vi "ArrayInRunTIme.vi"() -> ()   [LabVIEW 2019]
panel:
  in  "Array 2":dbl[](array[numeric])
  out "appended array":dbl[](array[numeric])
  in  "c":dbl
  in  "b":dbl
  in  "a":dbl
  out "initialized array":dbl[](array[numeric])
  in  "Array":dbl[](array[numeric])
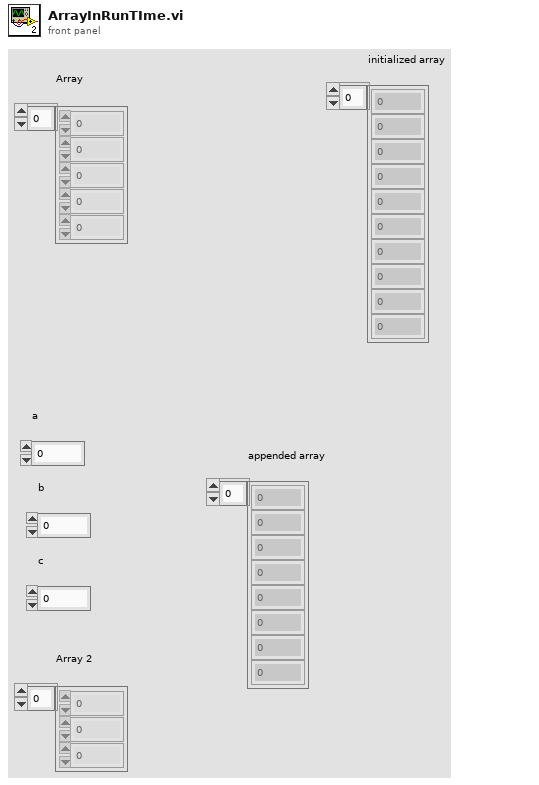
[diagram p1: front panel]
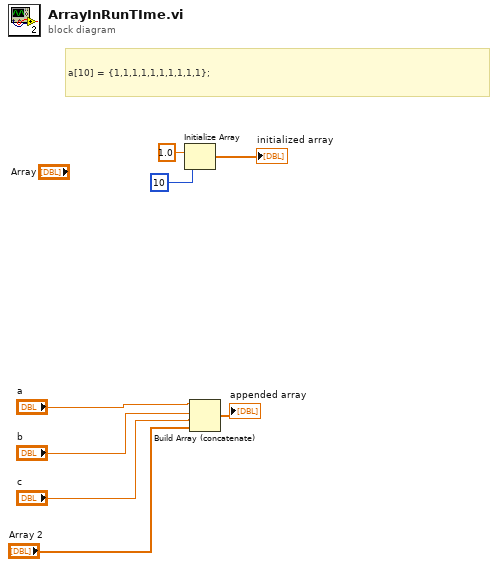
[diagram p0: block diagram]
diagram:
  # "a[10] = {1,1,1,1,1,1,1,1,1,1};"
  n1 = Initialize Array(1.0 ("element"), 10 ("dimension size")) -> (→"initialized array":dbl[])
  n2 = Build Array (concatenate)("a", "b", "c", "Array 2") -> (→"appended array":dbl[])
